vi "setUp.vi"(8 "error in (no error)":errorcluster, 11 "reference in":refnum<class "[Test Case] Put and Get file.lvclass">) -> (0 "error out":errorcluster, 3 "reference out":refnum<class "[Test Case] Put and Get file.lvclass">)   [LabVIEW 2015, in "Tests.lvlib" / "[Test Case] Put and Get file.lvclass"]
doc: "setUp runs prior to the test method during test execution. Use this method to initialize any object data required by your tests."
uses:
  [Test Case] Put and Get file.lvclass
  [Test Case] Put and Get file.lvclass/[Test Case] Put and Get file.ctl
  classes/File Transfer Behavior/File Transfer Behavior.lvclass/File Transfer Behavior.ctl
  classes/File Transfer Behavior/Get Password.vi
  classes/File Transfer Behavior/Get Username.vi
  classes/File Transfer Behavior/Get Address.vi
  classes/File Transfer Behavior/File Transfer Behavior.lvclass
  <vilib>/addons/_JKI Toolkits/VI Tester/TestCase.llb/TestCase.lvclass
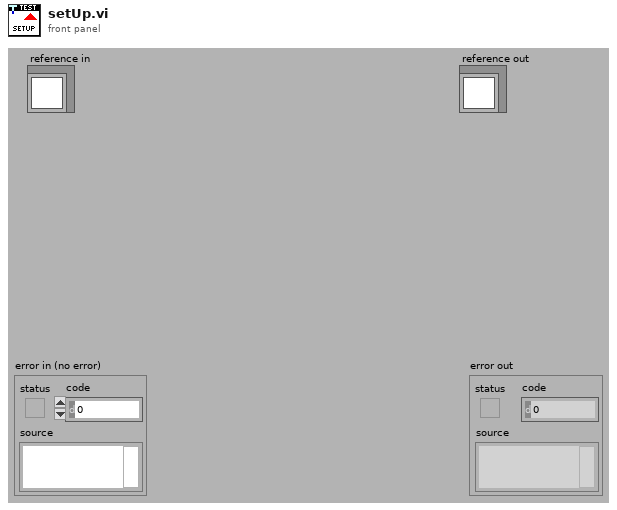
[diagram p1: front panel]
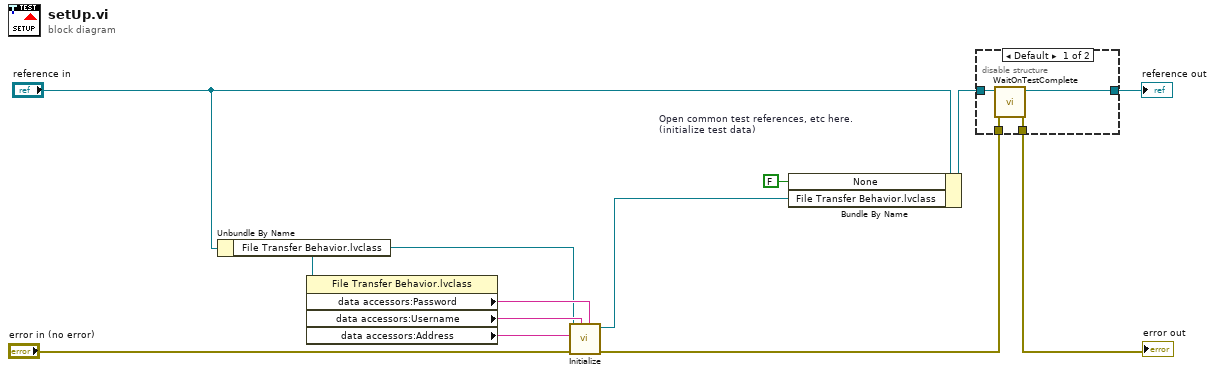
[diagram p0: block diagram]
diagram:
  w9 = FALSE  # Open common test references, etc here. (initialize test data)
  n1 = Unbundle By Name("reference in") -> ("File Transfer Behavior.lvclass"=w5:refnum<class "File Transfer Behavior.lvclass">)
  n2 = property class="File Transfer Behavior.lvclass"(reference=w5) -> ("data accessors:Password"=w8:string, "data accessors:Username"=w7:string, "data accessors:Address"=w6:string)  [unwired: 1 in, 2 out]
  n3 = call-dynamic "Initialize.vi"("Password"=w8, "Username"=w7, "error in (no error)"="error in (no error)", "Address"=w6, "File Transfer Behavior in"=w5) -> ("error out"=w2:errorcluster, "File Transfer Behavior out"=w3:refnum<class "File Transfer Behavior.lvclass">)  [unwired: 5 in]
  n4 = Bundle By Name(cluster="reference in", "None"=w9, "File Transfer Behavior.lvclass"=w3) -> (w10:refnum<class "[Test Case] Put and Get file.lvclass">)
  n5 = disable-structure shown="Default" {
    disable-tunnel: w2 -> [w16 w17]
    disable-tunnel: [w15 w17] -> w12
    disable-tunnel: [w14 w18] -> w11
    disable-tunnel: w10 -> [w13 w18]
    frame condition #0 (active) {
      n6 = call <vilib>:"WaitOnTestComplete.vi"("error in (no error)"=w16, "TestCase in"=w13) -> ("error out"=w15:errorcluster, "TestCase out"=w14:refnum<class "[Test Case] Put and Get file.lvclass">)  [unwired: 8 in]
    }
    frame condition #1 {
    }
  }
  "error out" <- w12
  "reference out" <- w11
